vi "emi_Defer Panel Updates OFF.vi"(5 "VI Refnum(This VI)":refnum<vi>, 9 "error in (no error)":errorcluster) -> (6 "VI Refnum Out":refnum<vi>, 10 "error out":errorcluster)   [LabVIEW 2011]
doc: "Gets a vi panel refrence, sets defere panel update to true, close panel refrence.\n\nIf not VI Refnum in, the refrence of the vi where this funciton is used is employed, and subsequently closed. (If refrence not explisitly vired, it does not need to be closed)\n\nIf error in: Perform action anyway\nIf error Still tries to turn off defere panel up date, if this generates error, it is put in Error out if no other error."
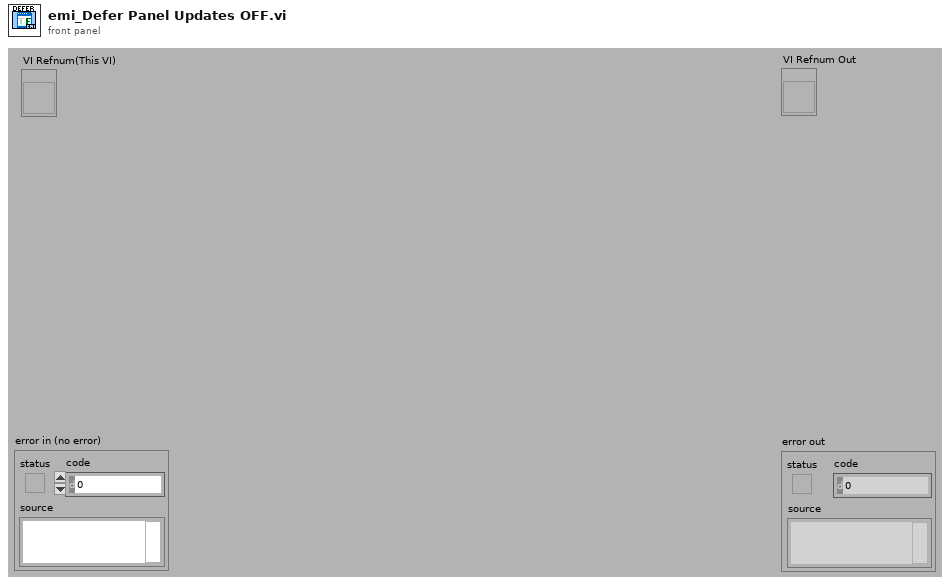
[diagram p1: front panel]
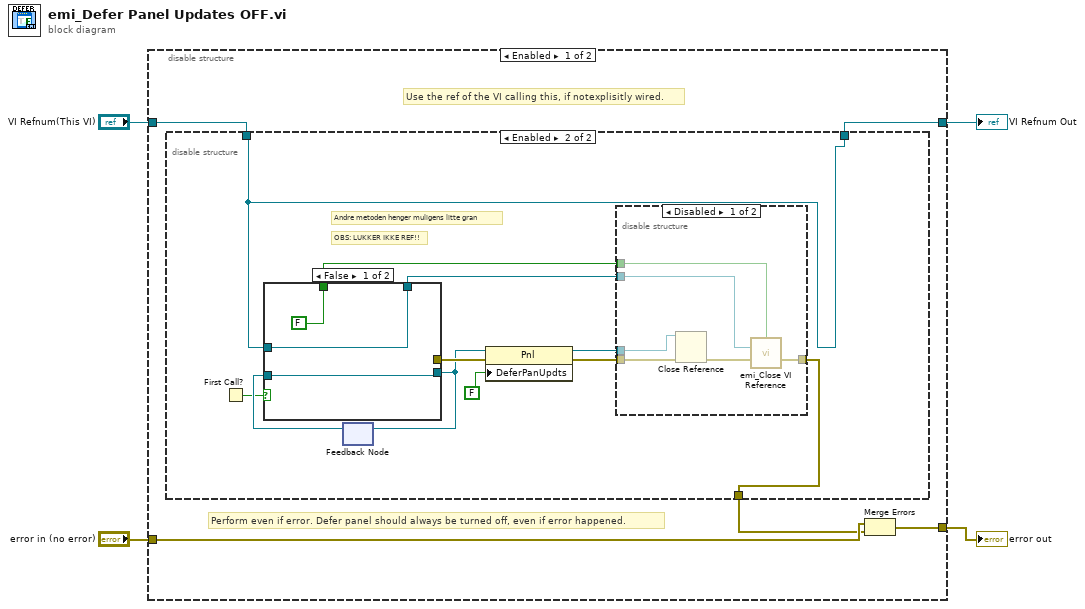
[diagram p0: block diagram]
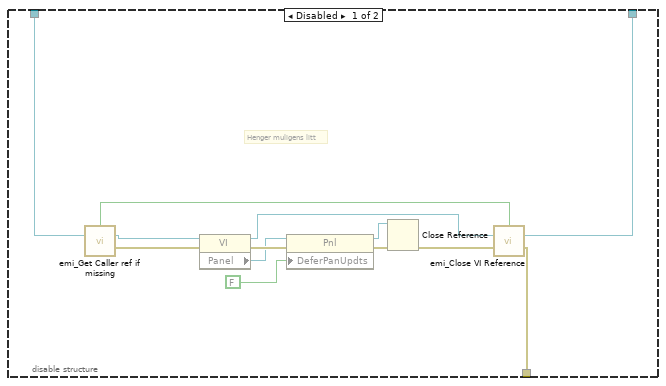
[diagram p2: hidden frame]
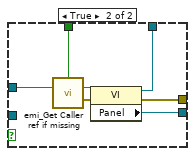
[diagram p3: hidden frame]
diagram:
  n1 = disable-structure shown="Enabled" {
    disable-tunnel: [w9 w52] -> w4
    disable-tunnel: "error in (no error)" -> [w8 w52]
    disable-tunnel: "VI Refnum(This VI)" -> [w6 w51]
    disable-tunnel: [w5 w51] -> w1
    frame Enabled {
      # "Perform even if error. Defer panel should always be turned off, even if error happened."
      # "Use the ref of the VI calling this, if notexplisitly wired."
      n2 = disable-structure shown="Enabled" {
        disable-tunnel: [w16 w23] -> w7
        disable-tunnel: w6 -> [w13 w24]
        disable-tunnel: [w12 w24] -> w5
        frame Disabled {
          # "Henger muligens litt"
          n3 = call "emi_Get Caller ref if missing.vi"("VI Refnum(Calling VI)"=w13) -> ("Ref Generated"=w17:bool, "VI Refnum Out"=w11:refnum<vi>, "error out"=w14:errorcluster)  [unwired: 12 in]
          n4 = property class="VI"(reference=w11, error in=w14) -> (reference out=w10:refnum<vi>, error out=w21:errorcluster, "Panel"=w20:refnum<vi>)
          n5 = property class="Pnl"(reference=w20, error in=w21, "DeferPanUpdts"=FALSE ("Defer Panel Updates")) -> (reference out=w19:refnum<vi>, error out=w18:errorcluster)
          n6 = Close Reference(reference=w19, error in (no error)=w18) -> (error out=w15:errorcluster)
          n7 = call "emi_Close VI Reference.vi"("Close ref?(T)"=w17, "VI Refnum"=w10, "error in (no error)"=w15) -> ("VI Refnum Out"=w12:refnum<vi>, "error out"=w16:errorcluster)  [unwired: 11 in]
        }
        frame Enabled {
          # "OBS: LUKKER IKKE REF!!"
          # "Andre metoden henger muligens litte gran"
          n8 = First Call?() -> (First Call?: T/F=w25:bool)
          n9 = feedback #1() -> (w26:refnum<vi>)  [unwired: 1 in]
          n10 = case shown="False" w25 {
            tunnel: [_ w43] -> w32
            tunnel: [w36 w42] -> w27
            tunnel: [FALSE ("Ref Generated") w41] -> w29
            tunnel: [w35 w38] -> w28
            tunnel: w24 -> [w35 w37]
            tunnel: w26 -> [w36 _]
            frame False {
            }
            frame True {
              n11 = call "emi_Get Caller ref if missing.vi"("VI Refnum(Calling VI)"=w37) -> ("Ref Generated"=w41:bool, "VI Refnum Out"=w39:refnum<vi>, "error out"=w40:errorcluster)  [unwired: 12 in]
              n12 = property class="VI"(reference=w39, error in=w40) -> (reference out=w38:refnum<vi>, error out=w43:errorcluster, "Panel"=w42:refnum<vi>)
            }
          }
          n13 = feedback-in #1(w27) -> ()
          n14 = property class="Pnl"(reference=w27, error in=w32, "DeferPanUpdts"=FALSE ("Defer Panel Updates")) -> (reference out=w31:refnum<vi>, error out=w30:errorcluster)
          n15 = disable-structure shown="Disabled" {
            disable-tunnel: w31 -> [w49 _]
            disable-tunnel: w30 -> [w48 w50]
            disable-tunnel: w29 -> [w47 _]
            disable-tunnel: [w46 w50] -> w23
            disable-tunnel: w28 -> [w44 _]
            frame Disabled {
              n16 = Close Reference(reference=w49, error in (no error)=w48) -> (error out=w45:errorcluster)
              n17 = call "emi_Close VI Reference.vi"("Close ref?(T)"=w47, "VI Refnum"=w44, "error in (no error)"=w45) -> ("error out"=w46:errorcluster)  [unwired: 11 in, 1 out]
            }
            frame Enabled {
            }
          }
        }
      }
      n18 = Merge Errors(w8, w7) -> (w9:errorcluster)
    }
    frame Disabled {
    }
  }
  "error out" <- w4
  "VI Refnum Out" <- w1
